vi "test3.vi"() -> ()   [LabVIEW 2014]
uses:
  <vilib>/sound2/lvsound2.llb/Sound Data Format.ctl
  <vilib>/sound2/lvsound2.llb/Sound Output Set Volume (Single).vi
  <vilib>/sound2/lvsound2.llb/Sound Output Write (DBL Single).vi
  <vilib>/measure/NI_MABase.lvlib
panel:
  in  "volume":dbl=100.0
  out "String":string="press"
  in  "stop":bool
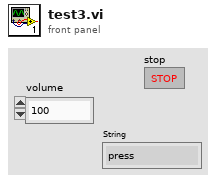
[diagram p1: front panel]
types:
  T1 = typedef "Sound Data Format.ctl" = cluster{"sample rate (S/s)":dbl, "number of channels":i32, "bits per sample":i32}
  T2 = typedef "Sound Output Task ID.ctl" = u32
  T3 = cluster{"sample rate (S/s)":dbl, "number of samples/ch":i32}
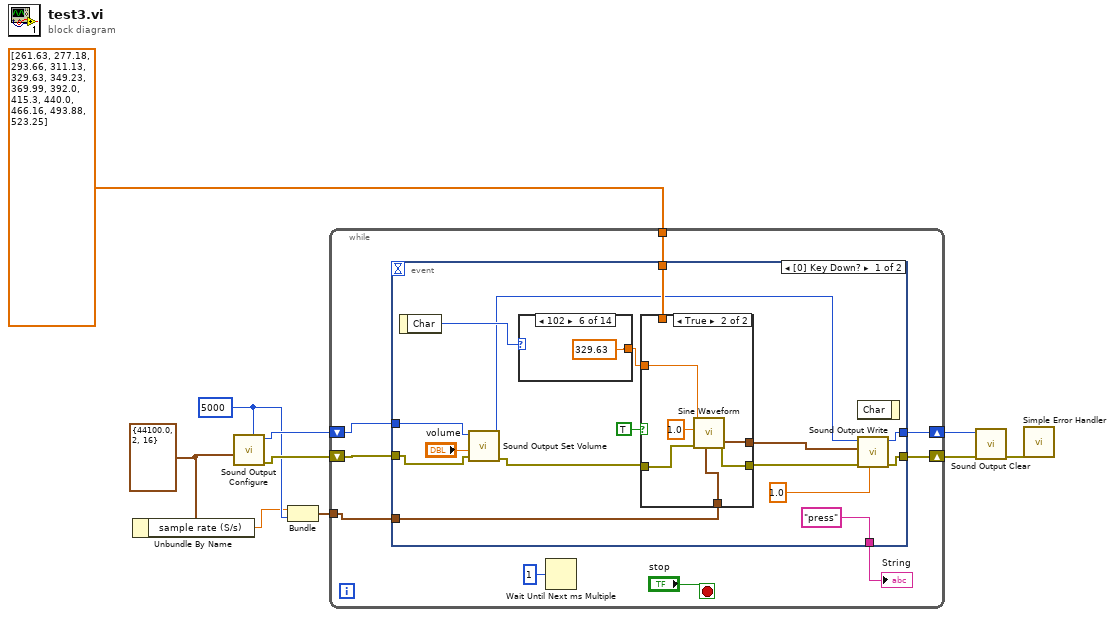
[diagram p0: block diagram]
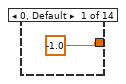
[diagram p3: hidden frame]
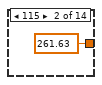
[diagram p4: hidden frame]
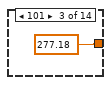
[diagram p5: hidden frame]
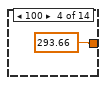
[diagram p6: hidden frame]
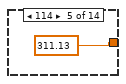
[diagram p7: hidden frame]
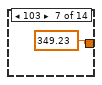
[diagram p8: hidden frame]
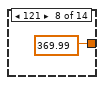
[diagram p9: hidden frame]
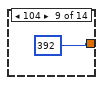
[diagram p10: hidden frame]
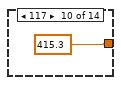
[diagram p11: hidden frame]
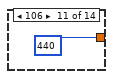
[diagram p12: hidden frame]
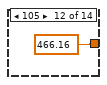
[diagram p13: hidden frame]
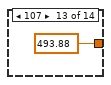
[diagram p14: hidden frame]
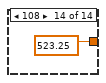
[diagram p15: hidden frame]
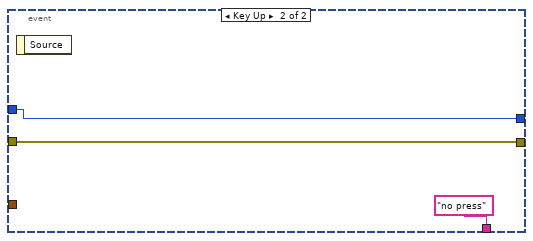
[diagram p16: hidden frame]
diagram:
  w7 = 5000 ("number of samples/ch")
  w8 = T1 {"sample rate (S/s)"=44100.0, "number of channels"=2, "bits per sample"=16} ("sound format")
  n1 = Unbundle By Name(w8) -> ("sample rate (S/s)"=w6:dbl)
  n2 = call <vilib>:"Sound Output Configure.vi"("number of samples/ch"=w7, "sound format"=w8) -> ("error out"=w9:errorcluster, "task ID"=w10:T2)  [unwired: 8 in]
  n3 = Bundle("sample rate (S/s)"=w6, "number of samples/ch"=w7) -> (w5:T3)  [unwired: 1 in]
  n4 = while {
    tunnel: w5 -> [w16]
    tunnel: dbl[] [261.63, 277.18, 293.66, 311.13, 329.63, 349.23, 369.99, 392.0, 415.3, 440.0, 466.16, 493.88, 523.25] -> [w17]
    shift-right: [w15] -> w4
    shift-left: w10 -> [w12]
    shift-right: [w14] -> w3
    shift-left: w9 -> [w11]
    stop <- "stop" stop-if-true
    n5 = event shown="[0] Key Down?" {
      selector: _ -> [_ _]
      dyn-events: _ -> [_ _]
      timeout: _ -> [_ _]
      tunnel: w17 -> [w31 _]
      tunnel: w16 -> [w30 _]
      tunnel: [w27 w59] -> w15
      tunnel: [w26 w58] -> w14
      tunnel: ["press" "no press"] -> w13
      tunnel: w12 -> [w23 w59]
      tunnel: w11 -> [w22 w58]
      event Key Down? {
        n6 = event-data() -> ("Char"=w35:i16)  [unwired: 1 in]
        n7 = call-poly <vilib>:"Sound Output Set Volume.vi"("error in (no error)"=w22, "volume"="volume", "task ID"=w23) -> ("error out"=w21:errorcluster, "task ID out"=w20:T2)  [unwired: 7 in]
        n8 = case shown="102" w35 {
          tunnel: [-1.0 261.63 277.18 293.66 311.13 329.63 349.23 369.99 392 415.3 440 466.16 493.88 523.25] -> w29
          frame 0, Default {
          }
          frame 115 {
          }
          frame 101 {
          }
          frame 100 {
          }
          frame 114 {
          }
          frame 102 {
          }
          frame 103 {
          }
          frame 121 {
          }
          frame 104 {
          }
          frame 117 {
          }
          frame 106 {
          }
          frame 105 {
          }
          frame 107 {
          }
          frame 108 {
          }
        }
        n9 = case shown="True" TRUE {
          tunnel: w21 -> [w36 w41]
          tunnel: [_ w40] -> w34
          tunnel: [w36 w39] -> w33
          tunnel: w30 -> [_ w38]
          tunnel: w31 -> [_ _]
          tunnel: w29 -> [_ w37]
          frame False {
          }
          frame True {
            n10 = call <vilib>:"Sine Waveform.vi"("sampling info"=w38, "error in (no error)"=w41, "amplitude"=1.0, "frequency"=w37) -> ("error out"=w39:errorcluster, "signal out"=w40:waveform(dbl))  [unwired: 6 in]
          }
        }
        n11 = event-data() -> ()  [unwired: 2 in, 1 out]
        n12 = call-poly <vilib>:"Sound Output Write.vi"("timeout (sec)"=1.0, "error in (no error)"=w33, "data"=w34, "task ID"=w20) -> ("error out"=w26:errorcluster, "task ID out"=w27:T2)  [unwired: 6 in]
      }
      event Key Up {
        n13 = event-data() -> ()  [unwired: 1 in, 1 out]
      }
    }
    "String" <- w13
    n14 = Wait Until Next ms Multiple(millisecond multiple=u32 1) -> ()  [unwired: 1 out]
  }
  n15 = call <vilib>:"Sound Output Clear.vi"("error in (no error)"=w3, "task ID"=w4) -> ("error out"=w2:errorcluster)  [unwired: 9 in]
  n16 = call <vilib>:"Simple Error Handler.vi"("error in (no error)"=w2) -> ()  [unwired: 4 in, 5 out]
